vi "GetPersistentConfiguration.vi"(8 "Error In":errorcluster, 9 "DataIn":variant, 11 "object in":refnum<class "YAFTAF.lvclass">) -> (0 "Error Out":errorcluster, 1 "DataOut":variant, 3 "object out":refnum<class "YAFTAF.lvclass">)   [LabVIEW 2021, in "YAFTAF.lvclass"]
uses:
  YAFTAF.lvclass
  C:/Localdata/Projects/TriekselSoft/TriekselsoftApplicationFramework/Source/.Externals/Library_YAF/YActor/YActor.lvclass
  YActor/YActor.lvclass/YActor.ctl
  YActor/ExeCmd_sync.vi
  YActor/private/SendCommand.vi
  YActor/private/WaitForReply.vi
  YActor/private/CreateLocalVI.vi
  YActor/private/ExeuteInlineVI.vi
  YActor/private/GetRemoteVIRef.vi
  YActor/private/GetNameOfVI.vi
  YActor/QuickCast.vi
  YActor/private/VINameProperty.vi
  YActor/private/MessageCounter.vi
  YActor/InlineReferencePool.vi
  YActor/private/ExecuteVI.vi
  YActor/YActor.lvclass
  C:/Localdata/Projects/TriekselSoft/TriekselsoftApplicationFramework/Source/.Externals/Interface_UserInterface_IFrontPanel/IFrontPanel/IFrontPanel.lvclass
  C:/Localdata/Projects/TriekselSoft/TriekselsoftApplicationFramework/Source/IInterface/IInterface.lvclass
  C:/Localdata/Projects/TriekselSoft/TriekselsoftApplicationFramework/Source/.Externals/Interface_Object_ICreateDestroy/ICreateDestroy/ICreateDestroy.lvclass
  C:/Localdata/Projects/TriekselSoft/TriekselsoftApplicationFramework/Source/.Externals/Interface_Object_IPersistentData/IPersistentData/IPersistentData.lvclass
  C:/Localdata/Projects/TriekselSoft/TriekselsoftApplicationFramework/Source/.Externals/Interface_TAF_ITAFObject/ITAFObject/ITAFObject.lvclass
  C:/Localdata/Projects/TriekselSoft/TriekselsoftApplicationFramework/Source/.Externals/Library_YAF/YAFTAF/YAFTAF.lvclass
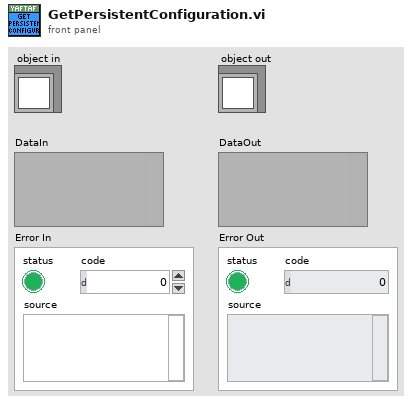
[diagram p1: front panel]
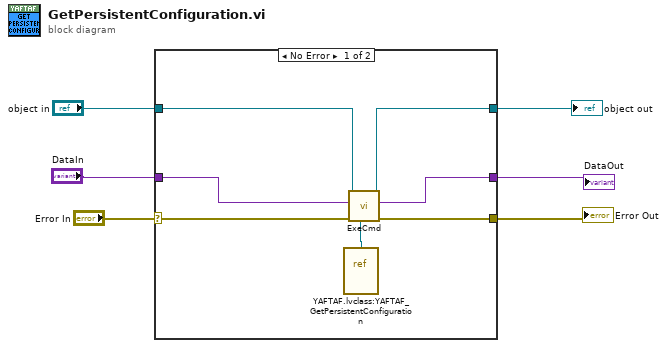
[diagram p0: block diagram]
diagram:
  n1 = case shown="No Error" "Error In" {
    selector: "Error In" -> [w8 w16]
    tunnel: [w13 w16] -> w2
    tunnel: [w11 w15] -> w4
    tunnel: "object in" -> [w9 w15]
    tunnel: "DataIn" -> [w7 w14]
    tunnel: [w10 w14] -> w3
    frame No Error {
      n2 = vi-ref "YAFTAF.lvclass:YAFTAF_GetPersistentConfiguration.vi"() -> (w12:refnum<vi>)
      n3 = call-poly "ExeCmd.vi"("CmdVIRef"=w12, "ErrorIn"=w8, "CmdData"=w7, "YActor in"=w9) -> ("ErrorOut"=w13:errorcluster, "ReplyData"=w10:variant, "YActor out"=w11:refnum<class "YAFTAF.lvclass">)  [unwired: 5 in]
    }
    frame Error {
    }
  }
  "Error Out" <- w2
  "object out" <- w4
  "DataOut" <- w3
